vi "Serialize.vi"(8 "error in (no error)":errorcluster, 11 "EXE Build in":refnum<class "LabVIEW Build.lvclass">) -> (0 "error out":errorcluster, 2 "Text":string)   [LabVIEW 2014, in "LabVIEW Build.lvclass"]
uses:
  LabVIEW Build.lvclass
  Shared/Controls/LabVIEW Build - STYP.ctl
  Classes/Job/Job.lvclass/Job.ctl
  LabVIEW Build.lvclass/LabVIEW Build.ctl
  Classes/Job/Read Executor Number.vi
  Classes/Job/Read WorkSpace Path.vi
  Read Auto Version Increment_.vi
  Read Project Path.vi
  Read Build Spec.vi
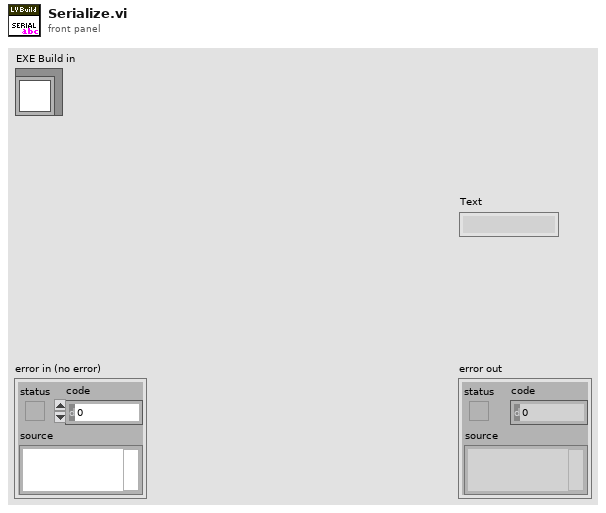
[diagram p1: front panel]
types:
  T1 = typedef "LabVIEW Build - STYP.ctl" = cluster{"Executor_Number":string, "Workspace_Path":string, "Build_Spec":string, "Target":string, "Project_Path":string, "Auto_Version_Increment":bool}
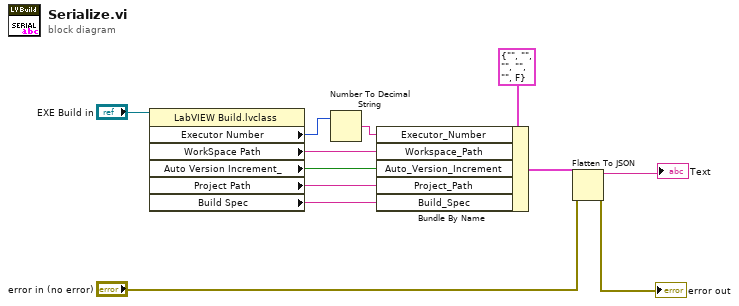
[diagram p0: block diagram]
diagram:
  n1 = property class="LabVIEW Build.lvclass"(reference="EXE Build in") -> ("Executor Number"=w2:i32, "WorkSpace Path"=w5:string, "Auto Version Increment_"=w7:bool, "Project Path"=w4:string, "Build Spec"=w6:string)  [unwired: 1 in, 2 out]
  n2 = Number To Decimal String(number=w2) -> (decimal integer string=w1:string)  [unwired: 1 in]
  n3 = Bundle By Name(cluster=T1 {"Executor_Number"="", "Workspace_Path"="", "Build_Spec"="", "Target"="", "Project_Path"="", "Auto_Version_Increment"=FALSE} ("EXE_Build"), "Executor_Number"=w1, "Workspace_Path"=w5, "Auto_Version_Increment"=w7, "Project_Path"=w4, "Build_Spec"=w6) -> (w8:T1)
  n4 = Flatten To JSON(anything=w8, error in (no error)="error in (no error)") -> (JSON string=→"Text":string, 11:→"error out":errorcluster)  [unwired: 1 in]
